vi "ScratchPad.vi"() -> ()   [LabVIEW 2013, in "Graph.lvclass"]
uses:
  Graph.lvclass
  <userlib>/_OpenG.lib/array/array.llb/Filter 1D Array__ogtk.vi
  <userlib>/_OpenG.lib/array/array.llb/Filter 1D Array (I32)__ogtk.vi
  <userlib>/_OpenG.lib/array/array.llb/Remove Duplicates from 1D Array__ogtk.vi
  <userlib>/_OpenG.lib/array/array.llb/Remove Duplicates from 1D Array (I32)__ogtk.vi
  <userlib>/_OpenG.lib/array/array.llb/Search Array__ogtk.vi
  <userlib>/_OpenG.lib/array/array.llb/Search 1D Array (I32)__ogtk.vi
  <userlib>/_OpenG.lib/array/array.llb/Delete Elements from Array__ogtk.vi
  <userlib>/_OpenG.lib/array/array.llb/Delete Elements from 1D Array (I32)__ogtk.vi
  <userlib>/_OpenG.lib/array/array.llb/Sort Array__ogtk.vi
  <userlib>/_OpenG.lib/array/array.llb/Sort 1D Array (I32)__ogtk.vi
  <userlib>/_OpenG.lib/array/array.llb/Reorder Array2__ogtk.vi
  <userlib>/_OpenG.lib/array/array.llb/Reorder 1D Array2 (I32)__ogtk.vi
panel:
  out "Paths DFS":i32[][](array[numeric])
  out "paths":i32[][](array[numeric])
  out "error out":errorcluster
  in  "error in (no error)":errorcluster
  out "values":variant[](array[variant])
  out "names":string[](array[string])
  out "Starting Vertices":i32[](array[numeric])
  out "Unique Values of Dictionary":i32[](array[numeric])
  out "variant out":variant
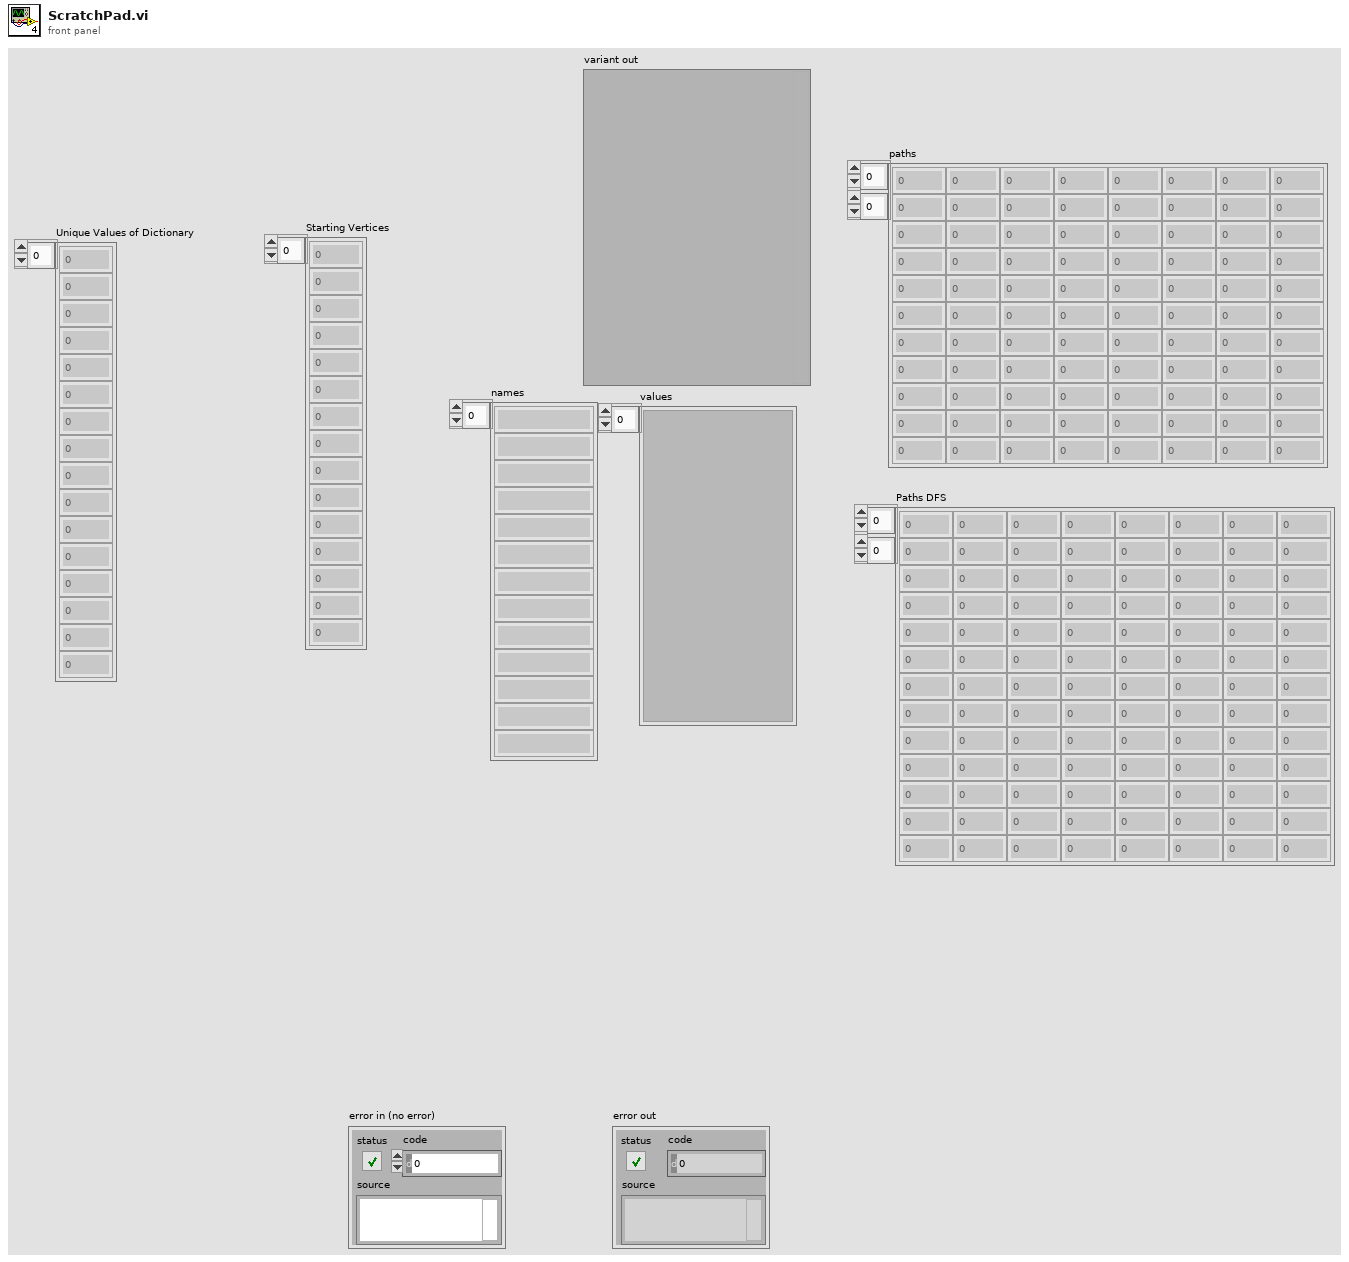
[diagram p1: front panel]
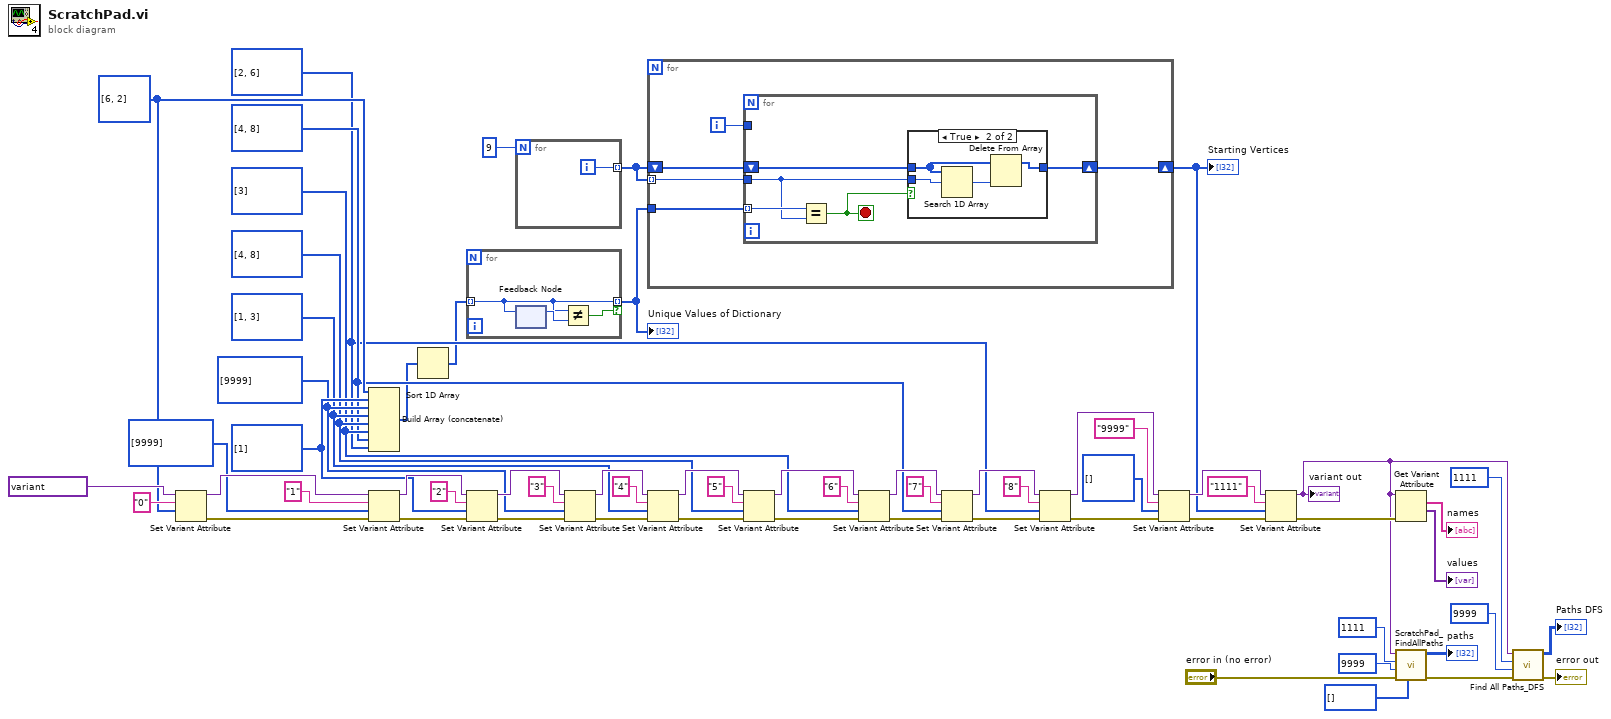
[diagram p0: block diagram]
diagram:
  w24 = i32[] [2, 6]
  w25 = i32[] [4, 8]
  w26 = i32[] [3]
  w27 = i32[] [4, 8]
  w28 = i32[] [1, 3]
  w29 = i32[] [9999]
  w30 = i32[] [1]
  w31 = i32[] [6, 2]
  n1 = Set Variant Attribute(Variant=variant ("variant"), name="0", value=w31) -> (Variant out=w60:variant, error out=w59:errorcluster)  [unwired: 1 in, 1 out]
  n2 = Build Array (concatenate)(w31, w30, w29, w28, w27, w26, w25, w24) -> (w23:i32[])
  n3 = Set Variant Attribute(Variant=w60, name="1", value=i32[] [9999], error in=w59) -> (Variant out=w56:variant, error out=w55:errorcluster)  [unwired: 1 out]
  n4 = Sort 1D Array(array=w23) -> (sorted array=w22:i32[])
  n5 = for {
    tunnel: w22 -> [w64] mode=indexing
    tunnel: [w64] -> w20 mode=indexing if=w63
    n6 = feedback-in #1(w64) -> ()
    n7 = feedback #1() -> (w65:i32)  [unwired: 1 in]
    n8 = Not Equal?(x=w64, y=w65) -> (x != y?=w63:bool)
  }
  "Unique Values of Dictionary" <- w20
  n9 = Set Variant Attribute(Variant=w56, name="2", value=w30, error in=w55) -> (Variant out=w53:variant, error out=w51:errorcluster)  [unwired: 1 out]
  n10 = for {
    N: 9 -> [_]
    tunnel: [w66] -> w19 mode=indexing
    i -> [w66]
  }
  n11 = Set Variant Attribute(Variant=w53, name="3", value=w29, error in=w51) -> (Variant out=w50:variant, error out=w49:errorcluster)  [unwired: 1 out]
  n12 = for {
    tunnel: w20 -> [w71]
    tunnel: w19 -> [w70] mode=indexing
    shift-right: [w68] -> w15
    shift-left: w19 -> [w69]
    i -> [w67]
    n13 = for {
      tunnel: w71 -> [w76] mode=indexing
      tunnel: w70 -> [w72]
      shift-right: [w74] -> w68
      shift-left: w69 -> [w75]
      tunnel: w67 -> [_]
      stop <- w73 stop-if-true
      n14 = Equal?(x=w76, y=w72) -> (x = y?=w73:bool)
      n15 = case shown="True" w73 {
        tunnel: w75 -> [w77 w80]
        tunnel: [w77 w81] -> w74
        tunnel: w72 -> [_ w79]
        frame False {
        }
        frame True {
          n16 = Search 1D Array(1D array=w80, element=w79) -> (index of element=w78:i32)  [unwired: 1 in]
          n17 = Delete From Array(array=w80, index=w78) -> (array with subset deleted=w81:i32[])  [unwired: 1 in, 1 out]
        }
      }
    }
  }
  "Starting Vertices" <- w15
  n18 = Set Variant Attribute(Variant=w50, name="4", value=w28, error in=w49) -> (Variant out=w47:variant, error out=w46:errorcluster)  [unwired: 1 out]
  n19 = Set Variant Attribute(Variant=w47, name="5", value=w27, error in=w46) -> (Variant out=w43:variant, error out=w44:errorcluster)  [unwired: 1 out]
  n20 = Set Variant Attribute(Variant=w43, name="6", value=w26, error in=w44) -> (Variant out=w41:variant, error out=w40:errorcluster)  [unwired: 1 out]
  n21 = Set Variant Attribute(Variant=w41, name="7", value=w25, error in=w40) -> (Variant out=w38:variant, error out=w37:errorcluster)  [unwired: 1 out]
  n22 = Set Variant Attribute(Variant=w38, name="8", value=w24, error in=w37) -> (Variant out=w35:variant, error out=w34:errorcluster)  [unwired: 1 out]
  n23 = Set Variant Attribute(Variant=w35, name="9999", value=i32[] [], error in=w34) -> (Variant out=w18:variant, error out=w17:errorcluster)  [unwired: 1 out]
  n24 = Set Variant Attribute(Variant=w18, name="1111", value=w15, error in=w17) -> (Variant out=w6:variant, error out=w14:errorcluster)  [unwired: 1 out]
  "variant out" <- w6
  n25 = Get Variant Attribute(Variant=w6, error in=w14) -> (names=→"names":string[], values=→"values":variant[])  [unwired: 2 in, 2 out]
  n26 = call "ScratchPad_FindAllPaths.vi"("path"=i32[] [], "error in (no error)"="error in (no error)", "End Vertex"=9999, "Start Vertex"=1111, "variant"=w6) -> ("error out"=w2:errorcluster, "paths"=→"paths":i32[][])  [unwired: 5 in]
  n27 = call "Find All Paths_DFS.vi"("error in (no error)"=w2, "End Vertex"=9999, "Start Vertex"=1111, "Graph Variant"=w6) -> ("error out"=→"error out":errorcluster, "Paths DFS"=→"Paths DFS":i32[][])  [unwired: 6 in]
